vi "Status Dichtheitstest.vi"(6 "Aktionen":T3, 7 "Protokoll":T1={"Startzeit"=timestamp(0 s since 1904-01-01), "Endzeit"=timestamp(0 s since 1904-01-01), "Startdruck"=0.0, "Enddruck"=0.0, "Dichtheitstest Umfang"=3} {"Dichtheitstest Umfang" items=["Pumpe / Filter / FT-IR / PNS", "Pumpe / Filter / FT-IR", "Filter / FT-IR", "FT-IR"]}, 8 "Fehler":bool, 9 "läuft?":bool, 10 "Anstieg":sgl, 11 "Zeitstempel":timestamp) -> (0 "Fehler":bool, 1 "läuft?":bool, 2 "Anstieg":sgl, 3 "Zeitstempel":timestamp, 5 "Protokoll":T1={"Startzeit"=timestamp(0 s since 1904-01-01), "Endzeit"=timestamp(0 s since 1904-01-01), "Startdruck"=0.0, "Enddruck"=0.0, "Dichtheitstest Umfang"=3} {"Dichtheitstest Umfang" items=["Pumpe / Filter / FT-IR / PNS", "Pumpe / Filter / FT-IR", "Filter / FT-IR", "FT-IR"]})   [LabVIEW 2020, in "Erweiterte Konfig.lvlib"]
uses:
  Erweiterte Konfig.lvlib
  Status Dichtheitstest Aktionen.ctl
  Dichtheitstest Protokoll.ctl
  Dichtheitstest Umfang.ctl
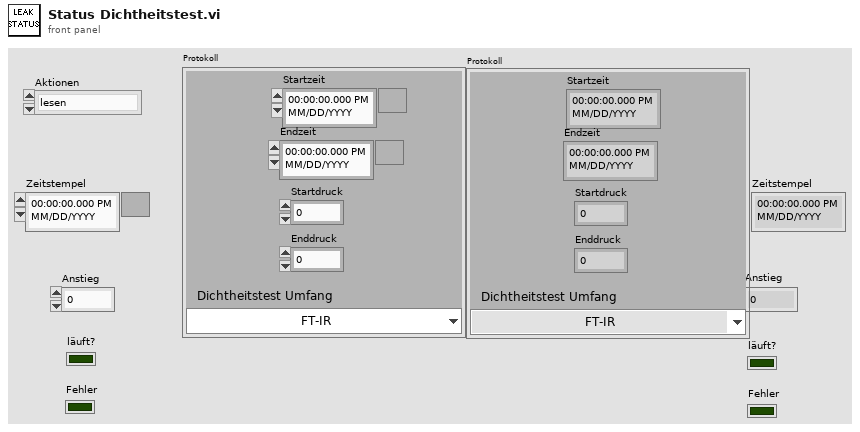
[diagram p1: front panel]
types:
  T1 = typedef "Erweiterte Konfig.lvlib/Dichtheitstest Protokoll.ctl" = cluster{"Startzeit":timestamp, "Endzeit":timestamp, "Startdruck":sgl, "Enddruck":sgl, "Dichtheitstest Umfang":T2}
  T2 = typedef "Erweiterte Konfig.lvlib/Dichtheitstest Umfang.ctl" = u16
  T3 = typedef "Erweiterte Konfig.lvlib/Status Dichtheitstest Aktionen.ctl" = enum16{"lesen", "Zeitstempel", "Daten", "läuft", "Protokolldaten"}
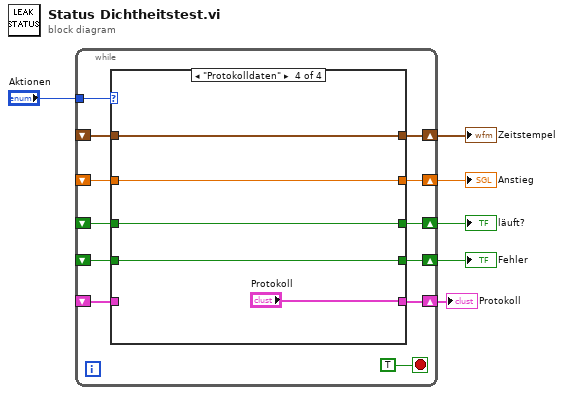
[diagram p0: block diagram]
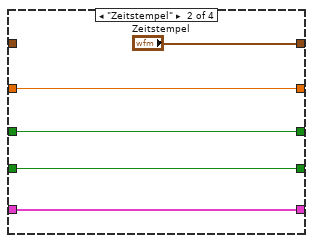
[diagram p3: hidden frame]
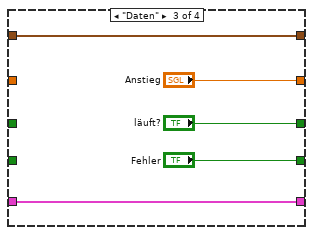
[diagram p4: hidden frame]
diagram:
  n1 = while {
    tunnel: "Aktionen" -> [w18]
    shift-right: [w17] -> w5
    shift-left: _ -> [w16]
    shift-right: [w14] -> w4
    shift-left: _ -> [w15]
    shift-right: [w12] -> w2
    shift-left: _ -> [w10]
    shift-right: [w11] -> w3
    shift-left: _ -> [w9]
    shift-right: [w8] -> w1
    shift-left: _ -> [w7]
    stop <- TRUE stop-if-true
    n2 = case shown="\"Protokolldaten\"" w18 {
      tunnel: [w23 "Zeitstempel" w32 w34] -> w17
      tunnel: w16 -> [w23 _ w32 w34]
      tunnel: w15 -> [w22 w27 _ w35]
      tunnel: [w22 w27 "Anstieg" w35] -> w14
      tunnel: [w21 w26 "läuft?" w36] -> w12
      tunnel: [w20 w25 "Fehler" w37] -> w11
      tunnel: w10 -> [w21 w26 _ w36]
      tunnel: w9 -> [w20 w25 _ w37]
      tunnel: [w19 w24 w29 "Protokoll"] -> w8
      tunnel: w7 -> [w19 w24 w29 _]
      frame "lesen", Default {
      }
      frame "Zeitstempel" {
      }
      frame "Daten" {
      }
      frame "Protokolldaten" {
      }
    }
  }
  "Zeitstempel" <- w5
  "Anstieg" <- w4
  "läuft?" <- w2
  "Fehler" <- w3
  "Protokoll" <- w1
